vi "TestExec.Config, Get Released SW Folder Info.vi"(8 "error in (no error)":errorcluster, 11 "Station Info":path) -> (0 "error out":errorcluster, 1 "Rel SW File":path, 2 "Seq Folder":path, 3 "Config Folder":path, 4 "SW Check En":bool, 5 "SW Check Int(s)":dbl)   [LabVIEW 2018]
uses:
  <vilib>/Utility/config.llb/Read Key (Path).vi
  <vilib>/Utility/config.llb/Read Key (Double).vi
  <vilib>/Utility/config.llb/Read Key (Boolean).vi
  <vilib>/Utility/config.llb/NI_LVConfig.lvlib
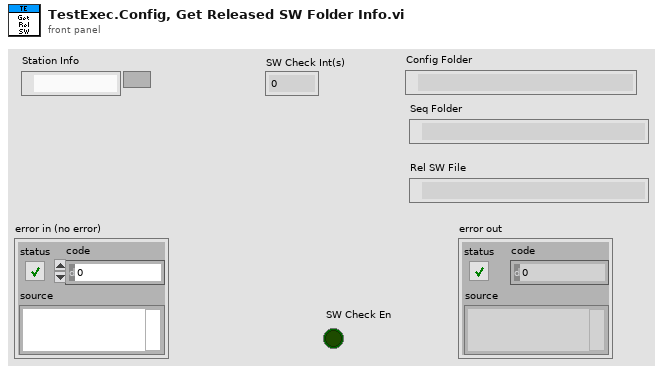
[diagram p1: front panel]
types:
  T1 = typedef "NI_LVConfig.lvlib/Config Data RefNum.ctl" = refnum<k1>
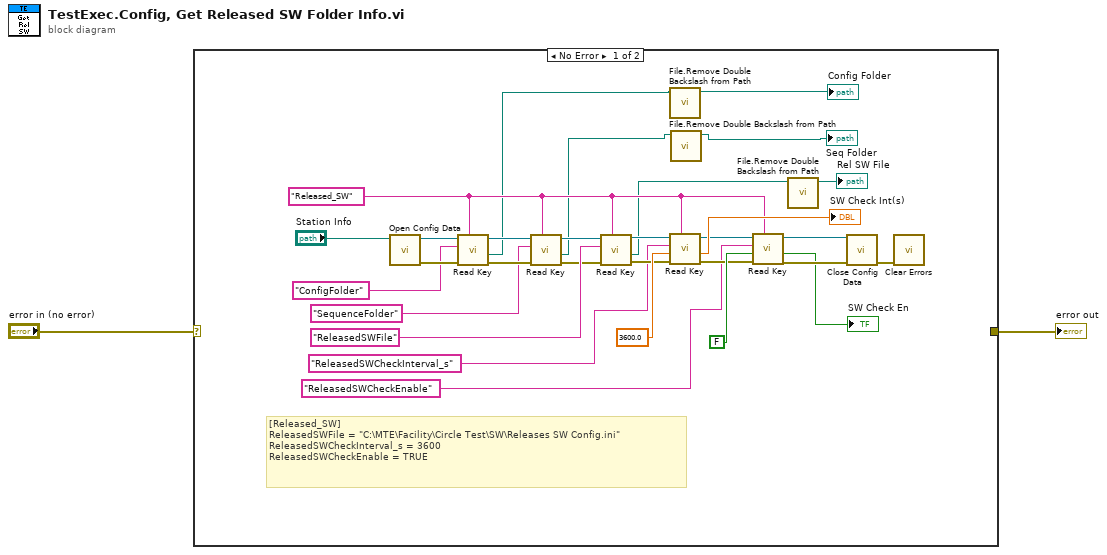
[diagram p0: block diagram]
diagram:
  n1 = case shown="No Error" "error in (no error)" {
    selector: "error in (no error)" -> [_ w33]
    tunnel: [_ w33] -> w1
    frame No Error {
      w13 = "Released_SW"
      # "[Released_SW]\nReleasedSWFile = \"C:\\MTE\\Facility\\Circle Test\\SW\\Releases SW Config.ini\"\nReleasedSWCheckInterval_s = 3600\nReleasedSWCheckEnable = TRUE"
      n2 = call <vilib>:"Open Config Data.vi"("configuration file path"="Station Info") -> ("error out"=w31:errorcluster, "refnum"=w32:T1)  [unwired: 8 in, 1 out]
      n3 = call-poly <vilib>:"Read Key.vi"("section"=w13, "error in (no error)"=w31, "key"="ConfigFolder", "refnum"=w32) -> ("error out"=w26:errorcluster, "value"=w6:path, "refnum out"=w27:T1)  [unwired: 4 in, 1 out]
      n4 = call-poly <vilib>:"Read Key.vi"("section"=w13, "error in (no error)"=w26, "key"="SequenceFolder", "refnum"=w27) -> ("error out"=w9:errorcluster, "value"=w7:path, "refnum out"=w23:T1)  [unwired: 4 in, 1 out]
      n5 = call-poly <vilib>:"Read Key.vi"("section"=w13, "error in (no error)"=w9, "key"="ReleasedSWFile", "refnum"=w23) -> ("error out"=w16:errorcluster, "value"=w8:path, "refnum out"=w24:T1)  [unwired: 4 in, 1 out]
      n6 = call "File.Remove Double Backslash from Path.vi"("Path"=w6) -> ("Path Out"=→"Config Folder":path)  [unwired: 10 in]
      n7 = call-poly <vilib>:"Read Key.vi"("section"=w13, "error in (no error)"=w16, "default value"=3600.0, "key"="ReleasedSWCheckInterval_s", "refnum"=w24) -> ("error out"=w17:errorcluster, "value"=→"SW Check Int(s)":dbl, "refnum out"=w19:T1)  [unwired: 3 in, 1 out]
      n8 = call "File.Remove Double Backslash from Path.vi"("Path"=w7) -> ("Path Out"=→"Seq Folder":path)  [unwired: 10 in]
      n9 = call-poly <vilib>:"Read Key.vi"("section"=w13, "error in (no error)"=w17, "default value"=FALSE, "key"="ReleasedSWCheckEnable", "refnum"=w19) -> ("error out"=w11:errorcluster, "value"=→"SW Check En":bool, "refnum out"=w12:T1)  [unwired: 3 in, 1 out]
      n10 = call "File.Remove Double Backslash from Path.vi"("Path"=w8) -> ("Path Out"=→"Rel SW File":path)  [unwired: 10 in]
      n11 = call <vilib>:"Close Config Data.vi"("error in (no error)"=w11, "refnum"=w12) -> ("error out"=w28:errorcluster)  [unwired: 8 in, 1 out]
      n12 = call <vilib>:"Clear Errors.vi"("error in (no error)"=w28) -> ()  [unwired: 5 in, 2 out]
    }
    frame Error {
    }
  }
  "error out" <- w1
